vi "Store Static VI References for Subpanel.vi"(8 "error in (no error)":errorcluster, 11 "HW Configuration in":refnum<class "HW Configuration.lvclass">) -> (0 "error out":errorcluster, 3 "HW Configuration out":refnum<class "HW Configuration.lvclass">)   [LabVIEW 2017, in "Hardware.lvlib" / "HW Configuration.lvclass"]
uses:
  HW Configuration.lvclass
  C:/Program Files (x86)/National Instruments/LabVIEW 2017/user.lib/Configuration Dialog Actor/Configuration.lvclass
  IO Mapping.vi
  <userlib>/Configuration Dialog Actor/Configuration.lvclass
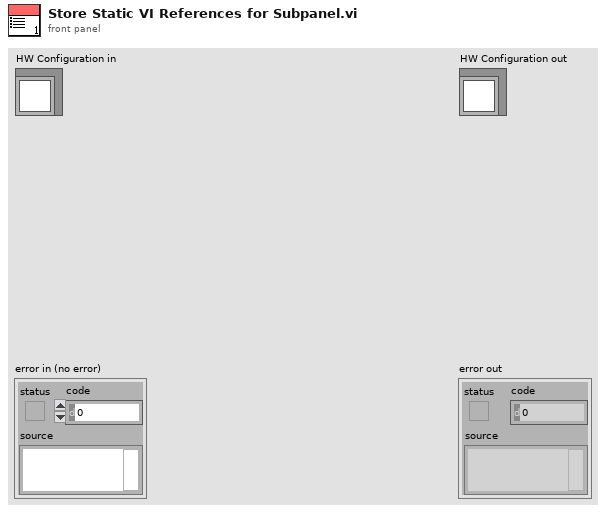
[diagram p1: front panel]
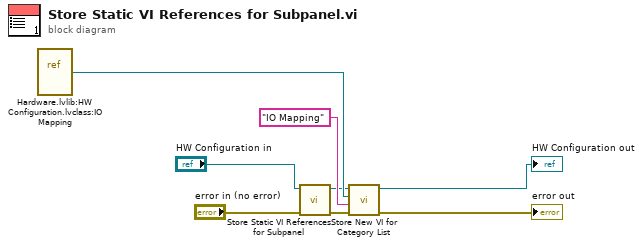
[diagram p0: block diagram]
diagram:
  n1 = vi-ref "Hardware.lvlib:HW Configuration.lvclass:IO Mapping.vi"() -> (w6:refnum<vi>)
  n2 = call-parent "Store Static VI References for Subpanel.vi"("error in (no error)"="error in (no error)", "Configuration in"="HW Configuration in") -> ("error out"=w2:errorcluster, "Configuration out"=w4:refnum<class "HW Configuration.lvclass">)  [unwired: 8 in]
  n3 = call <userlib>:"Store New VI for Category List.vi"("error in (no error)"=w2, "String"="IO Mapping", "VI Refnum"=w6, "Configuration in"=w4) -> ("error out"=→"error out":errorcluster, "Configuration out"=→"HW Configuration out":refnum<class "HW Configuration.lvclass">)  [unwired: 6 in]
